vi "file log variable.vi"(0 "memory usage":dbl, 1 "file name":string, 2 "X stage position":dbl, 3 "Y stage position":dbl, 4 "slice plane":dbl, 5 "error in":errorcluster, 6 "image plane":dbl, 7 "time":string, 8 "Item":T1=enum."X stage", 9 "Disk full space":dbl, 11 "Disk free space":dbl) -> (14 "output array":T2[](array[typedef]), 19 "error out":errorcluster)   [LabVIEW 2018]
uses:
  Controls/file log count.ctl
  Controls/file log.ctl
  Controls/file variable action.ctl
  Controls/FGV Actions.ctl
  Tile naming actions.ctl
panel:
  in  "file log count":T3
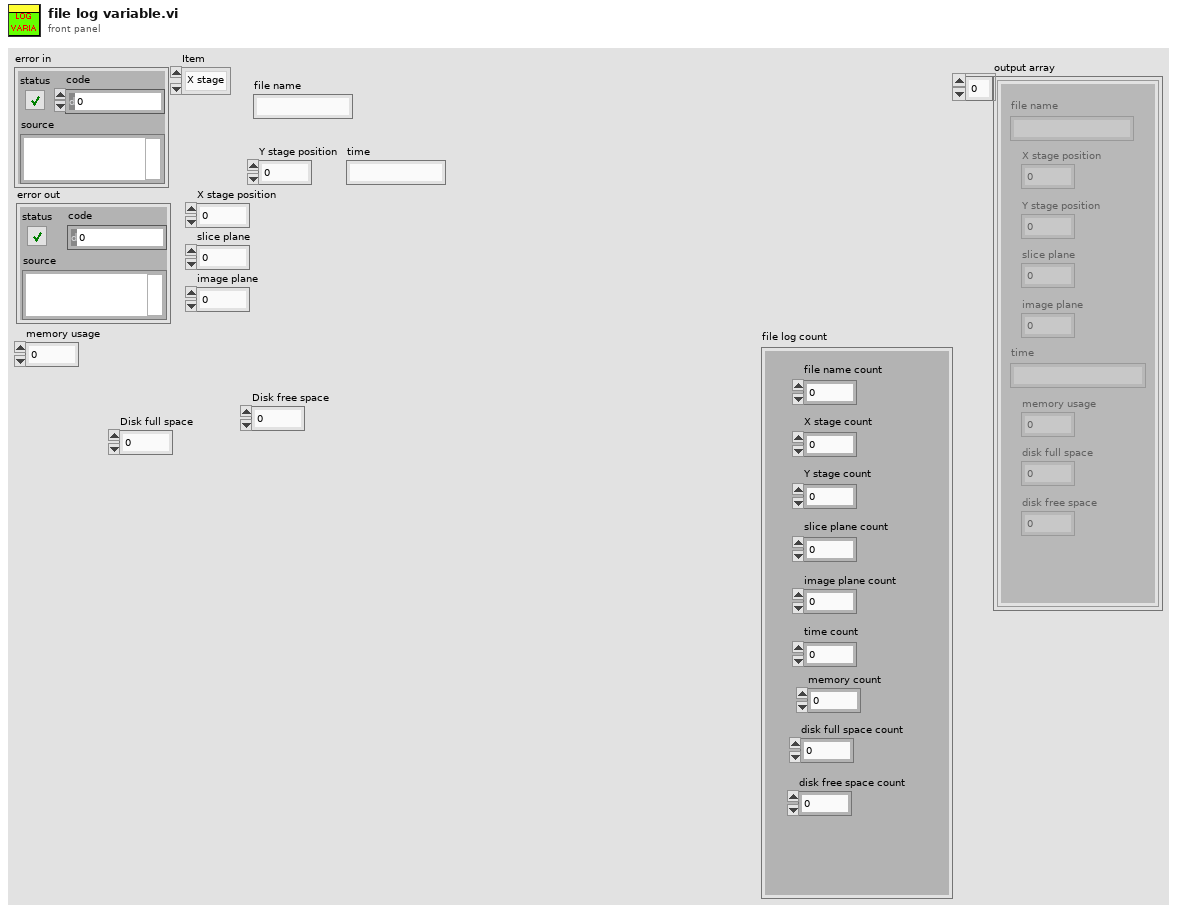
[diagram p1: front panel]
types:
  T1 = typedef "file variable action.ctl" = enum16{"File name", "X stage", "Y stage", "Slice plane", "Image plane", "time", "output", "Init", "Memory Usage", "Disk full Space", "Disk free space"}
  T2 = typedef "file log.ctl" = cluster{"file name":string, "X stage position":dbl, "Y stage position":dbl, "slice plane":dbl, "image plane":dbl, "time":string, "memory usage":dbl, "disk free space":dbl, "disk full space":dbl}
  T3 = typedef "file log count.ctl" = cluster{"time count":u32, "file name count":u32, "X stage count":u32, "Y stage count":u32, "slice plane count":u32, "image plane count":u32, "memory count":u32, "disk full space count":u32, "disk free space count":u32}
  T4 = typedef "Tile naming actions.ctl" = enum16{"Export", "Increment", "Total tile num", "Init"}
  T5 = typedef "FGV Actions.ctl" = enum16{"Init", "Set", "Get", "Clear"}
  T6 = typedef "System Parameters.ctl" = cluster{"Optical Parameters":T7, "Vibratome":T8, "Table Stages":T9, "Imaging Parameter":T12, "Galvo HW Parameters":cluster{"Analog Out Channel":tag, "Min Voltage":dbl, "Max Voltage":dbl, "Pixel Clock Source":tag, "Sample Rate":dbl, "Line Clock Out Ch":tag}, "Alazar parameters":T14, "Mosaic Paramter":cluster{"X Axis":cluster{"Start [mm]":dbl, "Steps [pts]":dbl, "End [mm]":dbl}, "Y Axis":cluster{"Start [mm]":dbl, "Steps [pts]":dbl, "End [mm]":dbl}, "Scan Pattern":enum16{"Uni-directional", "Bi-Directional", "Spiral Out", "Spiral In"}, "Overlap Options":cluster{"Overlap Type":enum16{"No Overlap", "X Only", "Y Only", "X and Y"}, "Percent Overlap":u8, "Justify":enum16{"Start", "Center", "End"}}}, "Manual Controls":T21, "Vibratome Axis":T24}
  T7 = typedef "Optical Parameters.ctl" = cluster{"Obj. Focal Length [mm]":dbl, "Scan Lens EFL[mm]":dbl, "Tube Lens EFL[mm]":dbl, "Galvo V Range (+/-)":dbl, "Galvo Max Half Angle [Deg]":dbl, "Max Galvo Range[%]":dbl}
  T8 = typedef "Vibratome Parameters.ctl" = cluster{"Z Bottom [mm]":dbl, "Pre Cut Dwell [s]":dbl, "Blade Frequency [RPM]":u16, "Slice Speed [mm/s]":dbl, "Post Cut Dwell [s]":dbl, "Ramp Time [s]":dbl, "Start X [mm]":dbl, "Start Y [mm]":dbl, "Slice Length [mm]":dbl, "Slice Axis":enum16{"X Axis", "Y Axis", "Z Axis"}, "Controller VISA Ref":refnum<visa-resource-name>}
  T9 = typedef "Translation Stage Parameters.ctl" = cluster{"X Stage":T10, "Y Stage":T10, "Z Stage":T10}
  T10 = typedef "Translation Stage Cluster.ctl" = cluster{"Position":dbl, "Is.Enabled?":bool, "Is.Connected?":bool, "Device SN":string, "AccelerationMaximum":dbl, "VelocityMaximum":dbl, "Acceleration":dbl, "Velocity":dbl, "waitTimeout (ms)":i32, "Model":T11, "Is.Homed?":bool}
  T11 = typedef "Translation Stage Types.ctl" = enum16{"None", "Thorlabs LTS", "Thorlabs MLJ"}
  T12 = typedef "Imaging Parameters.ctl" = cluster{"Raster Scan Direction":T13, "Pixel Dwell Time [Clock Cycles]":u16, "Flyback Time [Clock Cycles]":u16, "XY Center [um]":cluster{"X":dbl, "Y":dbl}, "Pixel Step Size [um] X":dbl, "XY Image Size":enum16{"32 x 32", "64 x 64", "128 x 128", "256 x 256", "512 x 512", "1024 x 1024", "2048 x 2048"}, "Custom":bool, "Custom Size":cluster{"X":u16, "Y":u16}, "Line Averages":u8, "Pixel Step Size [um] Y":dbl}
  T13 = typedef "Scan Direction.ctl" = enum16{"Uni Directional", "Bi Directional", "None"}
  T14 = typedef "Alazar parameters.ctl" = cluster{"Trigger Settings":cluster{"General Trigger Settings":T15, "Trigger Engine 1":T16, "Trigger Engine 2":T16}, "Device ID":T17, "Ch A Input Control":T18, "Ch B Input Control":T18, "Acq Settings":T19, "Capture Clock":T20}
  T15 = typedef "General Trigger Settings.ctl" = cluster{"Trigger Operation":u32, "Coupling ID":u32, "Range ID":u32, "Delay":u32, "Timeout Ticks":u32, "Mode":u32, "Parameter":u32}
  T16 = typedef "Trigger Engine Controls.ctl" = cluster{"Trigger Engine":u32, "Source":u32, "Slope":u32, "Level":u32}
  T17 = typedef "Alazar Device ID.ctl" = cluster{"System ID":u32, "Board ID":u32}
  T18 = typedef "Channel Input Controls.ctl" = cluster{"Channel":u8, "Coupling":u32, "Range":u32, "Impedance":u32}
  T19 = typedef "Alazar Acquisition Settings.ctl" = cluster{"Record Length":u32, "Offset":u32, "Records Per Buffer":u32, "Records Count (Records/Acq)":u32, "Window Type":u32, "Footer":u32, "Samples per record":u32, "Output Format":u32}
  T20 = typedef "Clock Controls.ctl" = cluster{"Sample Rate":u32, "Decimation":u32, "Source":u32, "Edge":u32}
  T21 = typedef "Manual Controls.ctl" = cluster{"Z0":dbl, "First image height":dbl, "Data Path":path, "Save parameters":T22, "Center Galvos":bool, "Acquisition mode":T23, "PSOCT Channel":u32, "Save":bool, "AIP rotation angle":dbl, "Scan Parameters":cluster{"# Scan":cluster{"#Ascan":i32, "#Bscan":i32}, "# Rpt":cluster{"#ARpt":i32, "#BRpt":i32}, "Aline Rate":u16, "# Extra":cluster{"# ARpt_extra":i32, "#Brtn_extra":i32}}, "ROI Parameters":cluster{"ROI (mm)":cluster{"X (mm)":dbl, "Y (mm)":dbl}, "Shift (mm)":cluster{"Xshift (mm)":sgl, "Yshift (mm)":sgl}}, "Objective":u16, "auto adjust focus":bool, "ret ds":bool}
  T22 = typedef "FFT parameters.ctl" = cluster{"start pixel":i32, "#pixels to save":i32}
  T23 = typedef "FFT mode.ctl" = enum16{"ThorOCT B line", "ThorOCT Spectral", "ThorOCT FFT", "Alazar B line", "Alazar FFT", "GPU FFT", "Alazar Spectral", "Simulation", "auto adjust focus"}
  T24 = typedef "Vibratome Param.ctl" = cluster{"Start [mm](first cut height)":dbl, "slice thickness[um]":dbl, "#slice":u16, "slice thick2[um]":dbl, "#thin slices":u16, "image thickness(um)":dbl, "#images":u16, "image depth2":dbl, "#image depth2":u16}
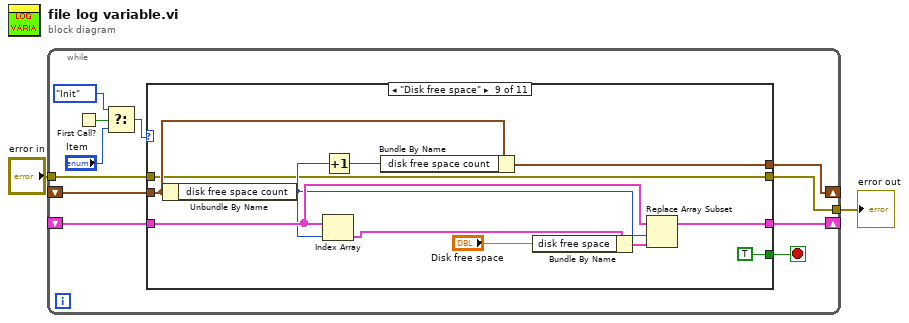
[diagram p0: block diagram]
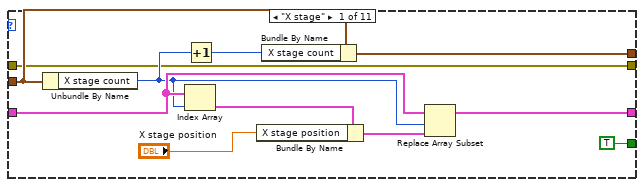
[diagram p2: hidden frame]
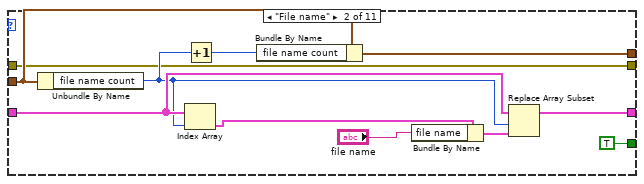
[diagram p3: hidden frame]
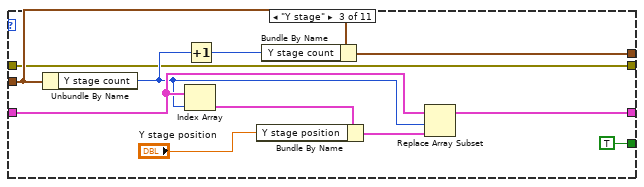
[diagram p4: hidden frame]
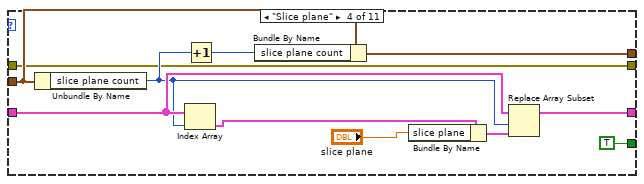
[diagram p5: hidden frame]
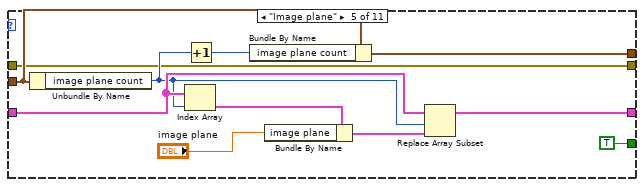
[diagram p6: hidden frame]
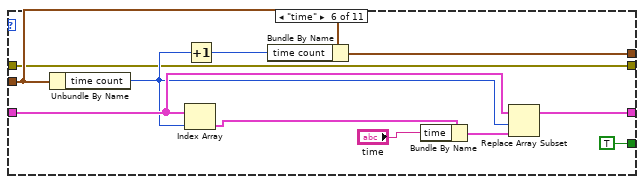
[diagram p7: hidden frame]
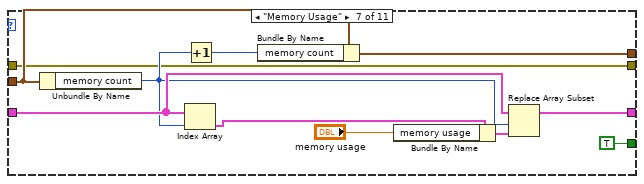
[diagram p8: hidden frame]
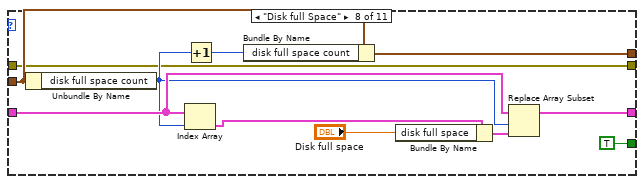
[diagram p9: hidden frame]
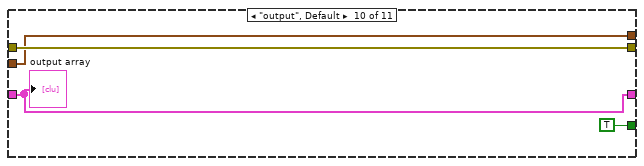
[diagram p10: hidden frame]
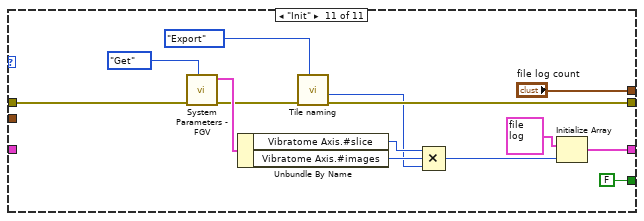
[diagram p11: hidden frame]
diagram:
  n1 = while {
    shift-right: [w12] -> _
    shift-left: _ -> [w13]
    shift-right: [w10] -> _
    shift-left: _ -> [w11]
    tunnel: "error in" -> [w9]
    tunnel: [w8] -> w1
    stop <- w7 stop-if-true
    n2 = First Call?() -> (First Call?: T/F=w5:bool)
    n3 = Select(t=file_variable_action."Init", s=w5, f="Item") -> (s? t:f=w3:T1)
    n4 = case shown="\"Disk free space\"" w3 {
      tunnel: w13 -> [w23 w34 w45 w56 w67 w78 w89 w100 w111 w114 _]
      tunnel: [w21 w32 w43 w54 w65 w76 w87 w98 w109 w114 w128] -> w12
      tunnel: w11 -> [w20 w31 w42 w53 w64 w75 w86 w97 w108 w115 _]
      tunnel: [w19 w30 w41 w52 w63 w74 w85 w96 w107 w115 "file log count"] -> w10
      tunnel: [w15 w26 w37 w48 w59 w70 w82 w93 w104 w116 w122] -> w8
      tunnel: w9 -> [w15 w26 w37 w48 w59 w70 w82 w93 w104 w116 w125]
      tunnel: [TRUE TRUE TRUE TRUE TRUE TRUE TRUE TRUE TRUE TRUE FALSE] -> w7
      frame "X stage" {
        n5 = Unbundle By Name(w20) -> ("X stage count"=w16:u32)
        n6 = Index Array(array=w23, index=w16) -> (element=w24:T2)
        n7 = Increment(x=w16) -> (x+1=w18:u32)
        n8 = Bundle By Name(cluster=w24, "X stage position"="X stage position") -> (w22:T2)
        n9 = Bundle By Name(cluster=w20, "X stage count"=w18) -> (w19:T3)
        n10 = Replace Array Subset(array=w23, new element=w22, index=w16) -> (w21:T2[])
      }
      frame "File name" {
        n11 = Unbundle By Name(w31) -> ("file name count"=w28:u32)
        n12 = Index Array(array=w34, index=w28) -> (element=w35:T2)
        n13 = Increment(x=w28) -> (x+1=w29:u32)
        n14 = Bundle By Name(cluster=w31, "file name count"=w29) -> (w30:T3)
        n15 = Bundle By Name(cluster=w35, "file name"="file name") -> (w33:T2)
        n16 = Replace Array Subset(array=w34, new element=w33, index=w28) -> (w32:T2[])
      }
      frame "Y stage" {
        n17 = Unbundle By Name(w42) -> ("Y stage count"=w39:u32)
        n18 = Index Array(array=w45, index=w39) -> (element=w46:T2)
        n19 = Increment(x=w39) -> (x+1=w40:u32)
        n20 = Bundle By Name(cluster=w46, "Y stage position"="Y stage position") -> (w44:T2)
        n21 = Bundle By Name(cluster=w42, "Y stage count"=w40) -> (w41:T3)
        n22 = Replace Array Subset(array=w45, new element=w44, index=w39) -> (w43:T2[])
      }
      frame "Slice plane" {
        n23 = Unbundle By Name(w53) -> ("slice plane count"=w49:u32)
        n24 = Index Array(array=w56, index=w49) -> (element=w57:T2)
        n25 = Increment(x=w49) -> (x+1=w51:u32)
        n26 = Bundle By Name(cluster=w53, "slice plane count"=w51) -> (w52:T3)
        n27 = Bundle By Name(cluster=w57, "slice plane"="slice plane") -> (w55:T2)
        n28 = Replace Array Subset(array=w56, new element=w55, index=w49) -> (w54:T2[])
      }
      frame "Image plane" {
        n29 = Unbundle By Name(w64) -> ("image plane count"=w60:u32)
        n30 = Index Array(array=w67, index=w60) -> (element=w68:T2)
        n31 = Increment(x=w60) -> (x+1=w62:u32)
        n32 = Bundle By Name(cluster=w64, "image plane count"=w62) -> (w63:T3)
        n33 = Bundle By Name(cluster=w68, "image plane"="image plane") -> (w66:T2)
        n34 = Replace Array Subset(array=w67, new element=w66, index=w60) -> (w65:T2[])
      }
      frame "time" {
        n35 = Unbundle By Name(w75) -> ("time count"=w71:u32)
        n36 = Index Array(array=w78, index=w71) -> (element=w79:T2)
        n37 = Increment(x=w71) -> (x+1=w73:u32)
        n38 = Bundle By Name(cluster=w75, "time count"=w73) -> (w74:T3)
        n39 = Bundle By Name(cluster=w79, "time"="time") -> (w77:T2)
        n40 = Replace Array Subset(array=w78, new element=w77, index=w71) -> (w76:T2[])
      }
      frame "Memory Usage" {
        n41 = Unbundle By Name(w86) -> ("memory count"=w83:u32)
        n42 = Index Array(array=w89, index=w83) -> (element=w90:T2)
        n43 = Increment(x=w83) -> (x+1=w84:u32)
        n44 = Bundle By Name(cluster=w86, "memory count"=w84) -> (w85:T3)
        n45 = Bundle By Name(cluster=w90, "memory usage"="memory usage") -> (w88:T2)
        n46 = Replace Array Subset(array=w89, new element=w88, index=w83) -> (w87:T2[])
      }
      frame "Disk full Space" {
        n47 = Unbundle By Name(w97) -> ("disk full space count"=w94:u32)
        n48 = Index Array(array=w100, index=w94) -> (element=w101:T2)
        n49 = Increment(x=w94) -> (x+1=w95:u32)
        n50 = Bundle By Name(cluster=w97, "disk full space count"=w95) -> (w96:T3)
        n51 = Bundle By Name(cluster=w101, "disk full space"="Disk full space") -> (w99:T2)
        n52 = Replace Array Subset(array=w100, new element=w99, index=w94) -> (w98:T2[])
      }
      frame "Disk free space" {
        n53 = Unbundle By Name(w108) -> ("disk free space count"=w105:u32)
        n54 = Index Array(array=w111, index=w105) -> (element=w112:T2)
        n55 = Increment(x=w105) -> (x+1=w106:u32)
        n56 = Bundle By Name(cluster=w108, "disk free space count"=w106) -> (w107:T3)
        n57 = Bundle By Name(cluster=w112, "disk free space"="Disk free space") -> (w110:T2)
        n58 = Replace Array Subset(array=w111, new element=w110, index=w105) -> (w109:T2[])
      }
      frame "output", Default {
        "output array" <- w114
      }
      frame "Init" {
        n59 = call "System Parameters - FGV.vi"("Actions"=FGV_Actions."Get", "Error In"=w125) -> ("Error Out"=w123:errorcluster, "System Parameters [Out]"=w126:T6)  [unwired: 8 in]
        n60 = Unbundle By Name(w126) -> ("Vibratome Axis.#slice"=w121:u16, "Vibratome Axis.#images"=w120:u16)
        n61 = call "Tile naming.vi"(7:Tile_naming_actions."Export", "Error In"=w123) -> ("Error Out"=w122:errorcluster, "Tile Num out"=w119:i32)  [unwired: 6 in, 2 out]
        n62 = Compound Arithmetic op=MULTIPLY(w121, w120, w119) -> (w118:i32)
        n63 = Initialize Array(T2 {"file name"="", "X stage position"=0.0, "Y stage position"=0.0, "slice plane"=0.0, "image plane"=0.0, "time"="", "memory usage"=0.0, "disk free space"=0.0, "disk full space"=0.0} ("File Log Array"), w118) -> (w128:T2[])
      }
    }
  }
  "error out" <- w1
